vi "switch_data_process.vi"   [LabVIEW 2016]
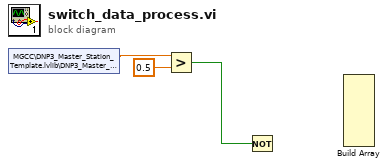
[diagram p0: block diagram]
diagram:
  n1 = shared-variable "MGCC\\DNP3_Master_Station_Template.lvlib\\DNP3_Master_Data_Variables.lvlib\\MS_Analog_Status.lvlib\\S0203-status"() -> (w2:dbl)  [unwired: 1 in, 1 out]
  n2 = Greater?(x=w2, y=0.5) -> (0:w1:bool)
  n3 = Not(x=w1) -> ()  [unwired: 1 out]
  n4 = Build Array() -> ()  [unwired: 9 in, 1 out]
